vi "main.vi"() -> ()   [LabVIEW 2015]
uses:
  Model/TestScenarioFactory/TestScenarioFactory/TestScenarioFactory.lvclass
  Model/TestLogFactory/TestLogFactory/TestLogFactory.lvclass
  Typedefs/TestLogTypes.ctl
  Typedefs/PassFailTest.ctl
  <userlib>/Common/Log/Config/Log.ctl
  Typedefs/TestExecution.ctl
  Model/TestLog/ITestLog/ITestLog.lvclass
  Model/TestScenario/ITestScenario/ITestScenario.lvclass
  Typedefs/ILCBTTypedefs.lvlib
  <userlib>/Common/ILC/ILC/ILC.lvclass
  <userlib>/Common/ConfigurationReader/ConfigurationReader.lvclass
  <userlib>/Common/Log/Log.lvlib
  ConfigurationThisComponent/ConfigurationThisComponent.lvclass
  ConfigurationTestParameters/ConfigurationTestParameters.lvclass
panel:
  in  "Interface Brd":string
  in  "Workstation":string
  in  "Edit Test Settings":bool
  in  "Edit Component Settings":bool
  out "Total Result":string
  out "Test Results":i32(listbox)
  out "Total Tests":i32
  out "Current Test Number":i32
  out "Currently Executing Test":string
  in  "Comments":string
  in  "Operator":string
  in  "Begin Testing":bool
  out "error out":errorcluster
  in  "Serial Number":string
  # "("
  # "of"
  # ")"
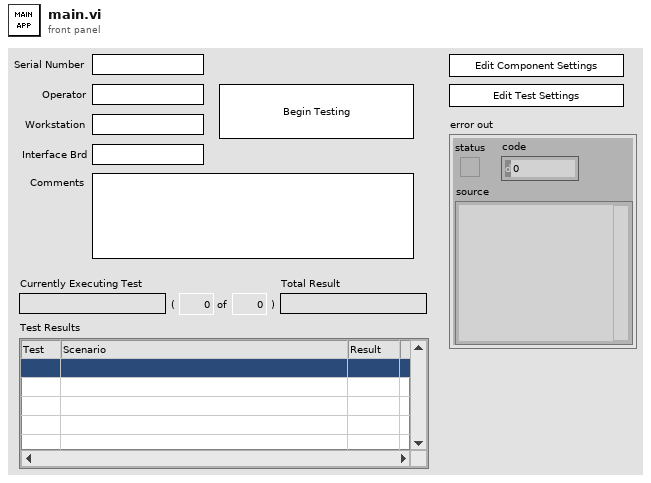
[diagram p1: front panel]
types:
  T1 = typedef "ILCBTTypedefs.lvlib/Test Settings.ctl" = cluster{"Collection Settings":T2, "TestExecutionOrder":T3, "Verify Voltage Tests":T5, "Verify DAC Tests":T7, "Set DAC Tests":T10, "Enable Disable":T12, "Pressure Tests":T13}
  T2 = typedef "ILCBTTypedefs.lvlib/Collection Settings.ctl" = cluster{"Samples To Average":i32, "Test Delay":dbl, "Linearity Step":i32}
  T3 = typedef "ILCBTTypedefs.lvlib/TestExecutionOrder.ctl" = T4[]
  T4 = typedef "ILCBTTypedefs.lvlib/TestScenarioTypes.ctl" = enum16{"+3.3VD", "+5.1V", "+24V", "RELVALV1", "RELVALV2", "Verify DAC_A = -1.00A", "Verify DAC_A = -0.75A", "Verify DAC_A = -0.50A", "Verify DAC_A = -0.25A", "Verify DAC_A = 0.00A", "Verify DAC_A = 0.25A", "Verify DAC_A = 0.50A", "Verify DAC_A = 0.75A", "Verify DAC_A = 1.00A", "Verify DAC_B = -1.00A", "Verify DAC_B = -0.75A", "Verify DAC_B = -0.50A", "Verify DAC_B = -0.25A", "Verify DAC_B = 0.00A", "Verify DAC_B = 0.25A", "Verify DAC_B = 0.50A", "Verify DAC_B = 0.75A", "Verify DAC_B = 1.00A", "Set DAC_A = -1.00A", "Set DAC_A = -0.75A", "Set DAC_A = -0.50A", "Set DAC_A = -0.25A", "Set DAC_A = 0.00A", "Set DAC_A = 0.25A", "Set DAC_A = 0.50A", "Set DAC_A = 0.75A", "Set DAC_A = 1.00A", "Set DAC_B = -1.00A", "Set DAC_B = -0.75A", "Set DAC_B = -0.50A", "Set DAC_B = -0.25A", "Set DAC_B = 0.00A", "Set DAC_B = 0.25A", "Set DAC_B = 0.50A", "Set DAC_B = 0.75A", "Set DAC_B = 1.00A", "Set MTR_PWR = On", "Set MTR_PWR = Off", "Set OUTPUT = On", "Set OUTPUT = Off", "Verify OUTPUT = On", "Verify OUTPUT = Off", "Verify POWER = Ok", "Verify POWER = Fail", "Verify AMP1 = Ok", "Verify AMP1 = Fail", "Verify AMP2 = Ok", "Verify AMP2 = Fail", "P1 0%", "P1 25%", "P1 50%", "P1 75%", "P1 100%", "P2 0%", "P2 25%", "P2 50%", "P2 75%", "P2 100%", "P3 0%", "P3 25%", "P3 50%", "P3 75%", "P3 100%", "P4 0%", "P4 25%", "P4 50%", "P4 75%", "P4 100%", "DCA 1 Linearity", "DCA 2 Linearity"}
  T5 = typedef "ILCBTTypedefs.lvlib/Verify Voltage Tests.ctl" = cluster{"+3.3VD":T6, "+5.1V":T6, "RELVALV1":T6, "RELVALV2":T6}
  T6 = typedef "ILCBTTypedefs.lvlib/Verify Voltage Test.ctl" = cluster{"DAQ Channel to Read":refnum<k21>, "Expected Value":dbl, "Tolerance":dbl}
  T7 = typedef "ILCBTTypedefs.lvlib/Verify DAC Tests.ctl" = cluster{"DAC A Channels":T8, "DAC B Channels":T8, "DAC = -1.00A":T9, "DAC = -0.75A":T9, "DAC = -0.50A":T9, "DAC = -0.25A":T9, "DAC = 0.00A":T9, "DAC = 0.25A":T9, "DAC = 0.50A":T9, "DAC = 0.75A":T9, "DAC = 1.00A":T9}
  T8 = typedef "ILCBTTypedefs.lvlib/DAC Channels.ctl" = cluster{"DAQ Channel 1 to Read":refnum<k21>, "DAQ Channel 2 to Read":refnum<k21>, "Resistor Ohms":dbl}
  T9 = typedef "ILCBTTypedefs.lvlib/Verify DAC Test.ctl" = cluster{"Expected Value":dbl, "Tolerance":dbl}
  T10 = typedef "ILCBTTypedefs.lvlib/Set DAC Tests.ctl" = cluster{"DAC = 0.00A":T11, "DAC = 0.25A":T11, "DAC = 0.5A":T11, "DAC = 0.75A":T11, "DAC = 1.0A":T11, "DAC = -0.25A":T11, "DAC = -0.5A":T11, "DAC = -0.75A":T11, "DAC = -1.0A":T11}
  T11 = typedef "ILCBTTypedefs.lvlib/Set DAC Test.ctl" = cluster{"Command Value":u16}
  T12 = typedef "ILCBTTypedefs.lvlib/Enable Disable.ctl" = cluster{"Motor Enable":u16, "Motor Disable":u16, "Current Output Enable":u16, "Current Output Disable":u16, "Power Enable":u16, "Power Disable":u16, "Amplifier Enable":u16, "Amplifier Disable":u16}
  T13 = typedef "ILCBTTypedefs.lvlib/Pressure Tests.ctl" = cluster{"0% Test":T14, "25% Test":T14, "50% Test":T14, "75% Test":T14, "100% Test":T14, "Settling (ms)":u16, "Delay (ms)":u16}
  T14 = typedef "ILCBTTypedefs.lvlib/Pressure Test.ctl" = cluster{"Command":u16, "Expected":u16, "Tolerance":u16}
  T15 = enum8{"Enabled", "Disabled", "Disabled and Grayed Out"}
  T16 = typedef "Log.lvlib/Log.ctl" = cluster{"Log Directory":path, "Log Filename Base":string, "Max records per file":u32, "Comment":string}
  T17 = typedef "ILCBTTypedefs.lvlib/PassFailTest.ctl" = enum16{"Fail", "Pass", "NA"}
  T18 = typedef "ILCBTTypedefs.lvlib/TestLogTypes.ctl" = enum16{"CSV Test Log"}
  T19 = typedef "ILCBTTypedefs.lvlib/TestExecution.ctl" = enum16{"Abort", "Continue"}
  T20 = typedef "LVRowAndColumnUnsignedTypeDef.ctl" = cluster{"Row":u32, "Column":u32}
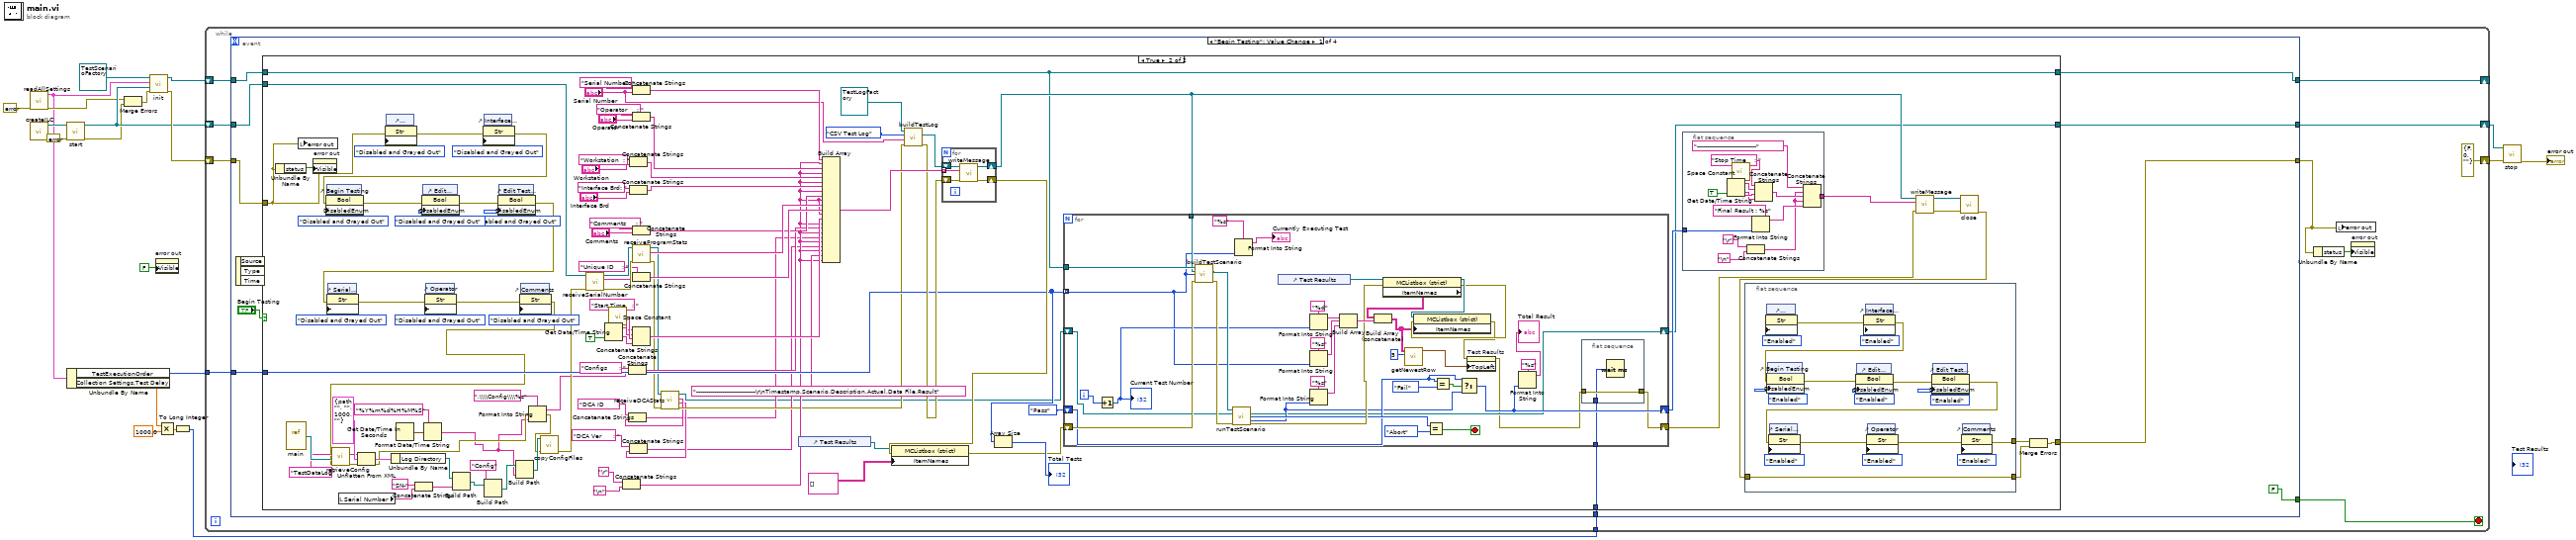
[diagram p0: block diagram]
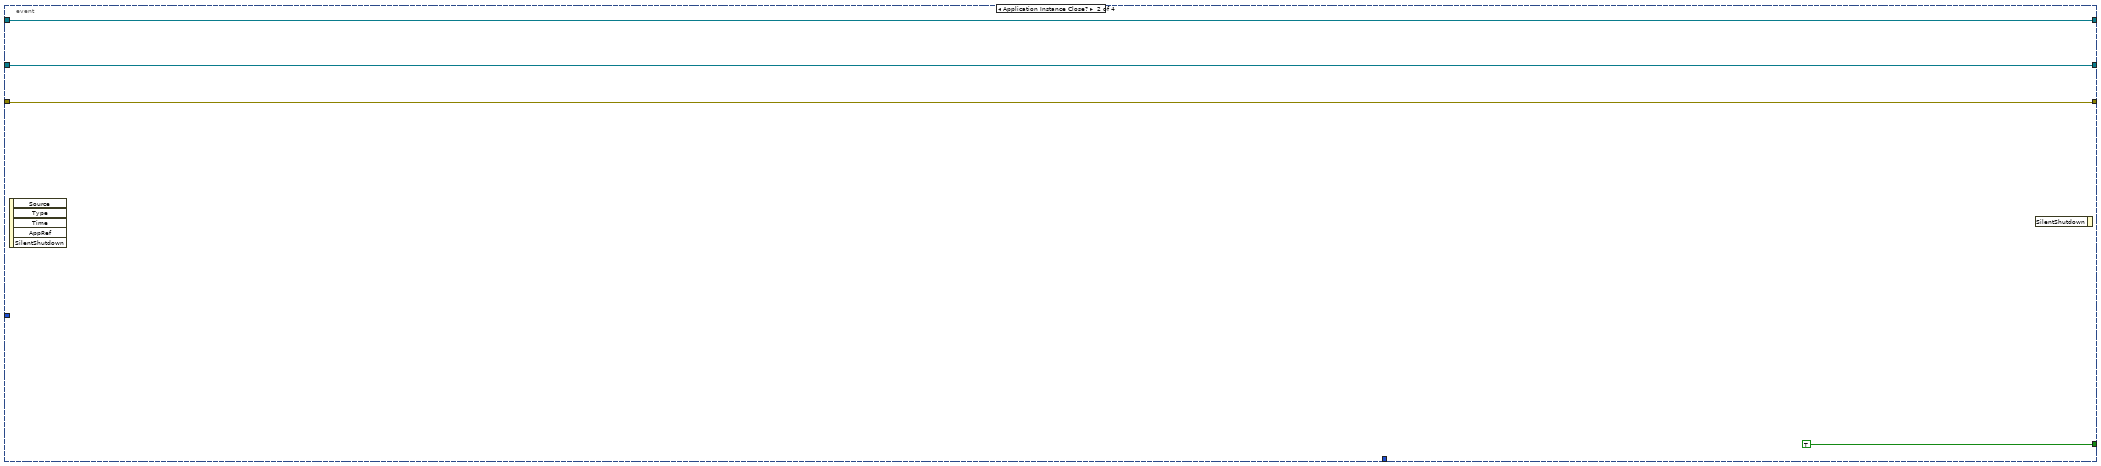
[diagram p3: hidden frame]
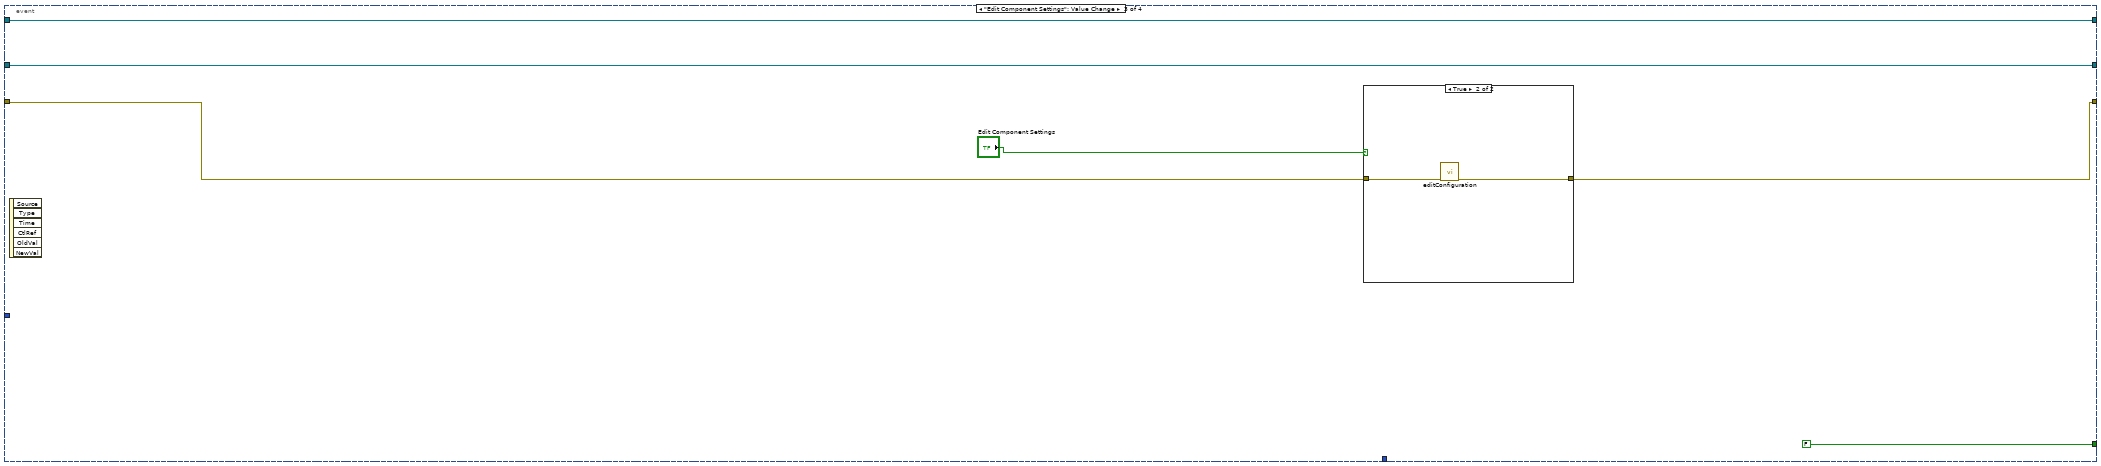
[diagram p4: hidden frame]
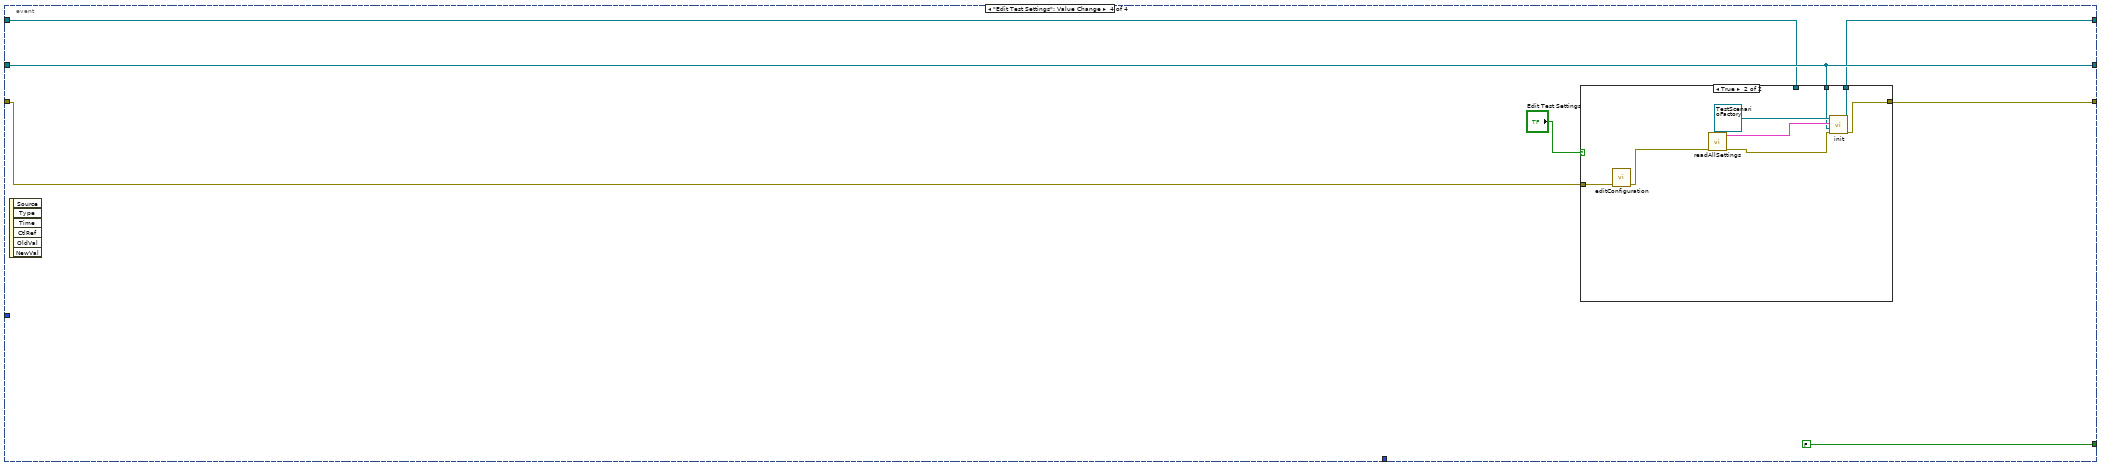
[diagram p6: hidden frame]
diagram:
  n1 = call "readAllSettings.vi"("error in (no error)"=errorcluster {"status"=FALSE, "code"=0, "source"=""}) -> ("error out"=w12:errorcluster, "ILC Settings"=w7:T1)  [unwired: 9 in]
  n2 = call "createILC.vi"() -> ("ILC"=w17:refnum<class "ILC.lvclass">)  [unwired: 11 in]
  n3 = call <userlib>:"start.vi"("error in (no error)"=errorcluster {"status"=FALSE, "code"=0, "source"=""}, "ILC in"=w17) -> ("error out"=w13:errorcluster, "ILC out"=w15:refnum<class "ILC.lvclass">)  [unwired: 8 in]
  n4 = Unbundle By Name(w7) -> ("TestExecutionOrder"=w6:T3, "Collection Settings.Test Delay"=w4:dbl)
  n5 = Merge Errors(w12, w13) -> (w14:errorcluster)
  n6 = call-dynamic "init.vi"("error in (no error)"=w14, "ILC"=w15, "ILC Settings"=w7, "TestScenarioFactory in"=refnum<class "TestScenarioFactory.lvclass"> refnum ("TestScenarioFactory.lvclass")) -> ("error out"=w18:errorcluster, "TestScenarioFactory out"=w19:refnum<class "TestScenarioFactory.lvclass">)  [unwired: 6 in]
  n7 = property on="error out" class="Clust (strict)"("Visible"=FALSE) -> ()  [unwired: 2 in, 2 out]
  n8 = Multiply(x=w4, y=1000.0) -> (x*y=w2:dbl)
  n9 = To Long Integer(number=w2) -> (32bit integer=w1:i32)
  n10 = while {
    shift-right: [w30] -> _
    shift-left: w19 -> [w31]
    shift-right: [errorcluster {"status"=FALSE, "code"=0, "source"=""} ("error out")] -> w10
    shift-left: w18 -> [w29]
    shift-right: [w27] -> w8
    shift-left: w15 -> [w28]
    tunnel: w6 -> [w26]
    tunnel: w1 -> [w21]
    stop <- w23 stop-if-true
    n11 = event shown="[0] \"Begin Testing\": Value Change" {
      selector: _ -> [_ _ _ _]
      dyn-events: _ -> [_ _ _ _]
      timeout: _ -> [_ _ _ _]
      tunnel: w31 -> [w37 w250 w255 w262]
      tunnel: [w37 w250 w255 w264] -> w30
      tunnel: [w34 w248 w256 w266] -> w25
      tunnel: w29 -> [w40 w248 w257 w267]
      tunnel: w28 -> [w39 w249 w254 w265]
      tunnel: [w38 w249 w254 w265] -> w27
      tunnel: w26 -> [w36 _ _ _]
      tunnel: [FALSE TRUE FALSE FALSE] -> w23
      tunnel: w21 -> [w32 _ _ _]
      event "Begin Testing": Value Change {
        n12 = event-data() -> ()  [unwired: 1 in, 3 out]
        n13 = case shown="True" "Begin Testing" {
          tunnel: w40 -> [w42 w59]
          tunnel: w39 -> [w41 w135]
          tunnel: [w41 w56] -> w38
          tunnel: w37 -> [w43 w71]
          tunnel: w36 -> [_ w116]
          tunnel: [w42 w72] -> w34
          tunnel: [w43 w71] -> _
          tunnel: w32 -> [_ w55]
          frame False {
          }
          frame True {
            n14 = Unbundle By Name(w59) -> ("status"=w70:bool)
            n15 = vi-ref "main.vi"() -> (w103:refnum<vi>)
            n16 = local write "error out"(w59) -> ()
            n17 = property on="error out" class="Clust (strict)"("Visible"=w70) -> ()  [unwired: 2 in, 2 out]
            n18 = control-ref of="Begin Testing"() -> (w160:refnum<vi>)
            n19 = control-ref of="Serial Number"() -> (w127:refnum<vi>)
            n20 = local read "Serial Number"() -> (w93:string)
            n21 = control-ref of="Workstation"() -> (w61:refnum<vi>)
            n22 = property class="Str"(reference=w61, error in=w59, "DisabledEnum"=T15."Disabled and Grayed Out" ("Disabled")) -> (error out=w63:errorcluster)  [unwired: 1 out]
            n23 = Get Date/Time In Seconds() -> (seconds since 1Jan1904=w106:timestamp)
            n24 = Concatenate Strings("SN-" ("string"), w93) -> (w91:string)
            n25 = control-ref of="Edit Component Settings"() -> (w86:refnum<vi>)
            n26 = Format Date/Time String(time format string (%c)="%Y%m%d%H%M%S", seconds (now)=w106) -> (date/time string=w76:string)  [unwired: 1 in]
            n27 = control-ref of="Operator"() -> (w126:refnum<vi>)
            n28 = control-ref of="Interface Brd"() -> (w62:refnum<vi>)
            n29 = property class="Str"(reference=w62, error in=w63, "DisabledEnum"=T15."Disabled and Grayed Out" ("Disabled")) -> (error out=w58:errorcluster)  [unwired: 1 out]
            n30 = property class="Bool"(reference=w160, error in=w58, "DisabledEnum"=T15."Disabled and Grayed Out" ("Disabled")) -> (error out=w87:errorcluster)  [unwired: 1 out]
            n31 = property class="Bool"(reference=w86, error in=w87, "DisabledEnum"=T15."Disabled and Grayed Out" ("Disabled")) -> (error out=w84:errorcluster)  [unwired: 1 out]
            n32 = control-ref of="Edit Test Settings"() -> (w81:refnum<vi>)
            n33 = property class="Bool"(reference=w81, error in=w84, "DisabledEnum"=T15."Disabled and Grayed Out" ("Disabled")) -> (error out=w83:errorcluster)  [unwired: 1 out]
            n34 = property class="Str"(reference=w127, error in=w83, "DisabledEnum"=T15."Disabled and Grayed Out" ("Disabled")) -> (error out=w122:errorcluster)  [unwired: 1 out]
            n35 = property class="Str"(reference=w126, error in=w122, "DisabledEnum"=T15."Disabled and Grayed Out" ("Disabled")) -> (error out=w121:errorcluster)  [unwired: 1 out]
            n36 = control-ref of="Comments"() -> (w123:refnum<vi>)
            n37 = property class="Str"(reference=w123, error in=w121, "DisabledEnum"=T15."Disabled and Grayed Out" ("Disabled")) -> (error out=w75:errorcluster)  [unwired: 1 out]
            n38 = call <userlib>:"retrieveConfig.vi"("error in (no error)"=w75, "callingVIRef"=w103, "configName"="TestDataLog") -> ("error out"=w95:errorcluster, "xmlData"=w104:string)  [unwired: 6 in, 1 out]
            n39 = Unflatten From XML(xml string=w104, type=T16 {"Log Directory"=path "", "Log Filename Base"="", "Max records per file"=1000, "Comment"=""} ("Log"), error in (no error)=w95) -> (value=w101:T16, error out=w77:errorcluster)
            n40 = Unbundle By Name(w101) -> ("Log Directory"=w94:path)
            n41 = Build Path(base path=w94, name or relative path=w91) -> (appended path=w80:path)
            n42 = Build Path(base path=w80, name or relative path="Config") -> (appended path=w79:path)
            n43 = Build Path(base path=w79, name or relative path=w76) -> (appended path=w97:path)
            n44 = Format Into String(format string=".\\\\Config\\\\%s", error in=w77, w76) -> (resulting string=w89:string, error out=w88:errorcluster)  [unwired: 1 in]
            n45 = call "copyConfigFiles.vi"("error in (no error)"=w88, "Destination"=w97) -> ("error out"=w96:errorcluster)  [unwired: 9 in]
            n46 = call <userlib>:"receiveSerialNumber.vi"("error in (no error)"=w96, "ILC in"=w135) -> ("error out"=w148:errorcluster, "Serial Number"=w142:string, "ILC out"=w147:refnum<class "ILC.lvclass">)  [unwired: 7 in]
            n47 = Get Date/Time String(want seconds? (F)=TRUE) -> (date string=w154:string, time string=w158:string)  [unwired: 2 in]
            n48 = call <vilib>:"Space Constant.vi"() -> ("String"=w155:string)
            n49 = Concatenate Strings("\r", "\n") -> (w54:string)
            n50 = Concatenate Strings("Configs      : " ("string"), w89) -> (w99:string)
            n51 = Concatenate Strings("Workstation  : " ("string"), "Workstation") -> (w67:string)
            n52 = Concatenate Strings("Interface Brd: " ("string"), "Interface Brd") -> (w66:string)
            n53 = Concatenate Strings("Serial Number: " ("string"), "Serial Number") -> (w149:string)
            n54 = Concatenate Strings("Operator     : " ("string"), "Operator") -> (w150:string)
            n55 = Concatenate Strings("Comments     : " ("string"), "Comments") -> (w151:string)
            n56 = call <userlib>:"receiveProgramStats.vi"("error in (no error)"=w148, "ILC in"=w147) -> ("error out"=w50:errorcluster, "Program Stats"=w152:string, "ILC out"=w51:refnum<class "ILC.lvclass">)  [unwired: 7 in]
            n57 = Concatenate Strings("Unique ID    : " ("string"), w142) -> (w153:string)
            n58 = Concatenate Strings("Start Time   : " ("string"), w154, w155, w158) -> (w157:string)
            n59 = call <userlib>:"receiveDCAStats.vi"("error in (no error)"=w50, "ILC in"=w51) -> ("error out"=w49:errorcluster, "Version"=w47:string, "Serial Number"=w48:string, "ILC out"=w44:refnum<class "ILC.lvclass">)  [unwired: 6 in]
            n60 = Concatenate Strings("DCA ID       : " ("string"), w48) -> (w45:string)
            n61 = Concatenate Strings("DCA Ver      : " ("string"), w47) -> (w46:string)
            n62 = control-ref of="Test Results"() -> (w117:refnum<vi>)
            n63 = Build Array(w149, w54, w150, w54, w67, w54, w66, w54, w151, w54, w152, w153, w54, w157, w54, w99, w54, w45, w54, w46, w54, "------------------------------\r\nTimestamp,Scenario,Description,Actual,Data File,Result", w54) -> (w138:string[])
            n64 = call-dynamic "buildTestLog.vi"("error in (no error)"=w49, "Serial Number"="Serial Number", "TestLogTypes"=TestLogTypes."CSV Test Log", "TestLogFactory in"=refnum<class "TestLogFactory.lvclass"> refnum ("TestLogFactory.lvclass")) -> ("error out"=w134:errorcluster, "ITestLog.lvclass"=w139:refnum<class "ITestLog.lvclass">)  [unwired: 5 in, 1 out]
            n65 = for {
              shift-right: [w243] -> w112
              shift-left: w139 -> [w246]
              tunnel: w138 -> [w245] mode=indexing
              shift-right: [w244] -> w119
              shift-left: w134 -> [w247]
              n66 = call-dynamic "writeMessage.vi"("error in (no error)"=w247, "Message"=w245, "ITestLog in"=w246) -> ("error out"=w244:errorcluster, "ITestLog out"=w243:refnum<class "ITestLog.lvclass">)  [unwired: 7 in]
            }
            n67 = property class="MCListbox (strict)"(reference=w117, error in=w119, "ItemNames"=string[][] []) -> (error out=w118:errorcluster)  [unwired: 1 out]
            n68 = Array Size(array=w116) -> (size(s)=→"Total Tests":i32)
            n69 = for {
              tunnel: w116 -> [w219] mode=indexing
              tunnel: w71 -> [w237]
              tunnel: w112 -> [w236]
              shift-right: [w201] -> w110
              shift-left: w118 -> [w238]
              shift-right: [w206] -> w113
              shift-left: PassFailTest."Pass" ("Result") -> [w213]
              shift-right: [w203] -> w56
              shift-left: w44 -> [w204]
              tunnel: w55 -> [w200]
              i -> [w233]
              stop <- w216 stop-if-true
              n70 = Increment(x=w233) -> (x+1=w220:i32)
              "Current Test Number" <- w220
              n71 = call-dynamic "buildTestScenario.vi"("TestScenarioFactory in"=w237, "Log"=w236, "Test Scenario"=w219, "error in (no error)"=w238) -> ("ITestScenario.lvclass"=w239:refnum<class "ITestScenario.lvclass">, "error out"=w240:errorcluster)  [unwired: 9 in, 1 out]
              n72 = call-dynamic "runTestScenario.vi"("ITestScenario in"=w239, "ILC"=w204, "error in (no error)"=w240) -> ("ILC 2"=w203:refnum<class "ILC.lvclass">, "TestExecution"=w218:T19, "Result"=w212:T17, "error out"=w222:errorcluster)  [unwired: 8 in, 1 out]
              n73 = Format Into String(format string="%s", w219) -> (resulting string=→"Currently Executing Test":string)  [unwired: 2 in, 1 out]
              n74 = control-ref of="Test Results"() -> (w232:refnum<vi>)
              n75 = Format Into String(format string="%d", w220) -> (resulting string=w227:string)  [unwired: 2 in, 1 out]
              n76 = Format Into String(format string="%s", w219) -> (resulting string=w228:string)  [unwired: 2 in, 1 out]
              n77 = Format Into String(format string="%s", w212) -> (resulting string=w229:string)  [unwired: 2 in, 1 out]
              n78 = Build Array(w227, w228, w229) -> (w230:string[])
              n79 = property class="MCListbox (strict)"(reference=w232, error in=w222) -> (reference out=w231:refnum<vi>, error out=w221:errorcluster, "ItemNames"=w223:string[][])
              n80 = Build Array (concatenate)(w223, w230) -> (w210:string[][])
              n81 = call "getNewestRow.vi"("Rows"=5, "Array"=w210) -> ("Top Left Visible Cell"=w209:T20)  [unwired: 9 in]
              n82 = property class="MCListbox (strict)"(reference=w231, error in=w221, "ItemNames"=w210) -> (error out=w211:errorcluster)  [unwired: 1 out]
              n83 = Equal?(x=w218, y=TestExecution."Abort") -> (x = y?=w216:bool)
              n84 = Equal?(x=w213, y=PassFailTest."Fail") -> (x = y?=w214:bool)
              n85 = Select(t=w213, s=w214, f=w212) -> (s? t:f=w206:T17)
              n86 = property on="Test Results" class="MCListbox (strict)"(error in=w211, "TopLeft"=w209) -> (error out=w202:errorcluster)  [unwired: 1 in, 1 out]
              n87 = Format Into String(format string="%s", w206) -> (resulting string=→"Total Result":string)  [unwired: 2 in, 1 out]
              n88 = flat-sequence {
                tunnel: w202 -> [w242]
                tunnel: [w242] -> w201
                tunnel: w200 -> [w241]
                frame #0 {
                  n89 = Wait (ms)(milliseconds to wait=w241) -> ()  [unwired: 1 out]
                }
              }
            }
            n90 = flat-sequence {
              tunnel: w113 -> [w188]
              tunnel: [w187] -> w107
              frame #0 {
                n91 = Get Date/Time String(want seconds? (F)=TRUE) -> (date string=w196:string, time string=w194:string)  [unwired: 2 in]
                n92 = call <vilib>:"Space Constant.vi"() -> ("String"=w195:string)
                n93 = Concatenate Strings("\r", "\n") -> (w186:string)
                n94 = Format Into String(format string="Final Result : %s", w188) -> (resulting string=w189:string)  [unwired: 2 in, 1 out]
                n95 = Concatenate Strings("Stop Time    : " ("string"), w196, w195, w194) -> (w190:string)
                n96 = Concatenate Strings("------------------------------", w186, w190, w186, w189) -> (w187:string)
              }
            }
            n97 = flat-sequence {
              tunnel: w108 -> [w167]
              tunnel: [w168] -> w73
              tunnel: [w167] -> w74
              frame #0 {
                n98 = control-ref of="Workstation"() -> (w162:refnum<vi>)
                n99 = property class="Str"(reference=w162, "DisabledEnum"=T15."Enabled" ("Disabled")) -> (error out=w166:errorcluster)  [unwired: 1 in, 1 out]
                n100 = control-ref of="Begin Testing"() -> (w178:refnum<vi>)
                n101 = control-ref of="Serial Number"() -> (w184:refnum<vi>)
                n102 = control-ref of="Edit Component Settings"() -> (w170:refnum<vi>)
                n103 = control-ref of="Interface Brd"() -> (w164:refnum<vi>)
                n104 = property class="Str"(reference=w164, error in=w166, "DisabledEnum"=T15."Enabled" ("Disabled")) -> (error out=w161:errorcluster)  [unwired: 1 out]
                n105 = property class="Bool"(reference=w178, error in=w161, "DisabledEnum"=T15."Enabled" ("Disabled")) -> (error out=w173:errorcluster)  [unwired: 1 out]
                n106 = property class="Bool"(reference=w170, error in=w173, "DisabledEnum"=T15."Enabled" ("Disabled")) -> (error out=w175:errorcluster)  [unwired: 1 out]
                n107 = control-ref of="Operator"() -> (w183:refnum<vi>)
                n108 = control-ref of="Edit Test Settings"() -> (w171:refnum<vi>)
                n109 = property class="Bool"(reference=w171, error in=w175, "DisabledEnum"=T15."Enabled" ("Disabled")) -> (error out=w172:errorcluster)  [unwired: 1 out]
                n110 = property class="Str"(reference=w184, error in=w172, "DisabledEnum"=T15."Enabled" ("Disabled")) -> (error out=w181:errorcluster)  [unwired: 1 out]
                n111 = property class="Str"(reference=w183, error in=w181, "DisabledEnum"=T15."Enabled" ("Disabled")) -> (error out=w180:errorcluster)  [unwired: 1 out]
                n112 = control-ref of="Comments"() -> (w177:refnum<vi>)
                n113 = property class="Str"(reference=w177, error in=w180, "DisabledEnum"=T15."Enabled" ("Disabled")) -> (error out=w168:errorcluster)  [unwired: 1 out]
              }
            }
            n114 = call-dynamic "writeMessage.vi"("error in (no error)"=w110, "Message"=w107, "ITestLog in"=w112) -> ("error out"=w109:errorcluster, "ITestLog out"=w111:refnum<class "ITestLog.lvclass">)  [unwired: 7 in]
            n115 = call-dynamic "close.vi"("error in (no error)"=w109, "ITestLog in"=w111) -> ("error out"=w108:errorcluster)  [unwired: 8 in, 1 out]
            n116 = Merge Errors(w73, w74) -> (w72:errorcluster)
          }
        }
      }
      event Application Instance Close? {
        n117 = event-data() -> ()  [unwired: 1 in, 5 out]
        n118 = event-data() -> ()  [unwired: 2 in, 1 out]
      }
      event "Edit Component Settings": Value Change {
        n119 = event-data() -> ()  [unwired: 1 in, 6 out]
        n120 = case shown="True" "Edit Component Settings" {
          tunnel: w257 -> [w258 w260]
          tunnel: [w258 w259] -> w256
          frame False {
          }
          frame True {
            n121 = call "editConfiguration.vi"("error in (no error)"=w260) -> ("error out"=w259:errorcluster)  [unwired: 9 in, 1 out]
          }
        }
      }
      event "Edit Test Settings": Value Change {
        n122 = event-data() -> ()  [unwired: 1 in, 6 out]
        n123 = case shown="True" "Edit Test Settings" {
          tunnel: w267 -> [w268 w277]
          tunnel: [w268 w272] -> w266
          tunnel: w265 -> [_ w271]
          tunnel: [w269 w270] -> w264
          tunnel: w262 -> [w269 _]
          frame False {
          }
          frame True {
            n124 = call "editConfiguration.vi"("error in (no error)"=w277) -> ("error out"=w274:errorcluster)  [unwired: 8 in, 2 out]
            n125 = call "readAllSettings.vi"("error in (no error)"=w274) -> ("error out"=w273:errorcluster, "ILC Settings"=w275:T1)  [unwired: 9 in]
            n126 = call-dynamic "init.vi"("error in (no error)"=w273, "ILC"=w271, "ILC Settings"=w275, "TestScenarioFactory in"=refnum<class "TestScenarioFactory.lvclass"> refnum ("TestScenarioFactory.lvclass")) -> ("error out"=w272:errorcluster, "TestScenarioFactory out"=w270:refnum<class "TestScenarioFactory.lvclass">)  [unwired: 6 in]
          }
        }
      }
    }
    n127 = Unbundle By Name(w25) -> ("status"=w24:bool)
    n128 = local write "error out"(w25) -> ()
    n129 = property on="error out" class="Clust (strict)"("Visible"=w24) -> ()  [unwired: 2 in, 2 out]
  }
  n130 = call <userlib>:"stop.vi"("error in (no error)"=w10, "ILC in"=w8) -> ("error out"=→"error out":errorcluster)  [unwired: 8 in, 1 out]
